vi "Control.vi"() -> ()   [LabVIEW 2024]
uses:
  <vilib>/Instr/_visa.llb/VISA Configure Serial Port (Instr).vi
panel:
  in  "OK Button":bool
  in  "Enter Speed":dbl(slide) scale=10.0..100.0
  in  "VISA resource name":refnum<visa-resource-name>
  in  "Stop Button":bool
  out "Boolean 4":bool
  out "Boolean 3":bool
  out "Boolean 2":bool
  out "Boolean":bool
  in  "Next Button":bool
  in  "Previous Button":bool
  in  "Down Button":bool
  in  "Up Button":bool
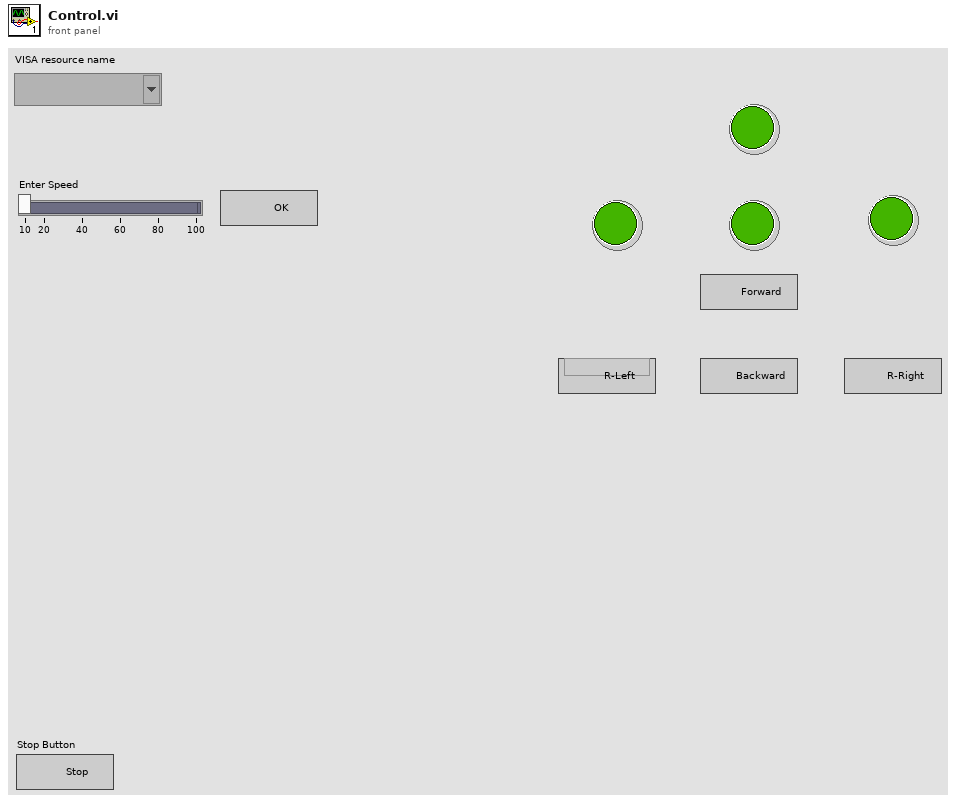
[diagram p1: front panel]
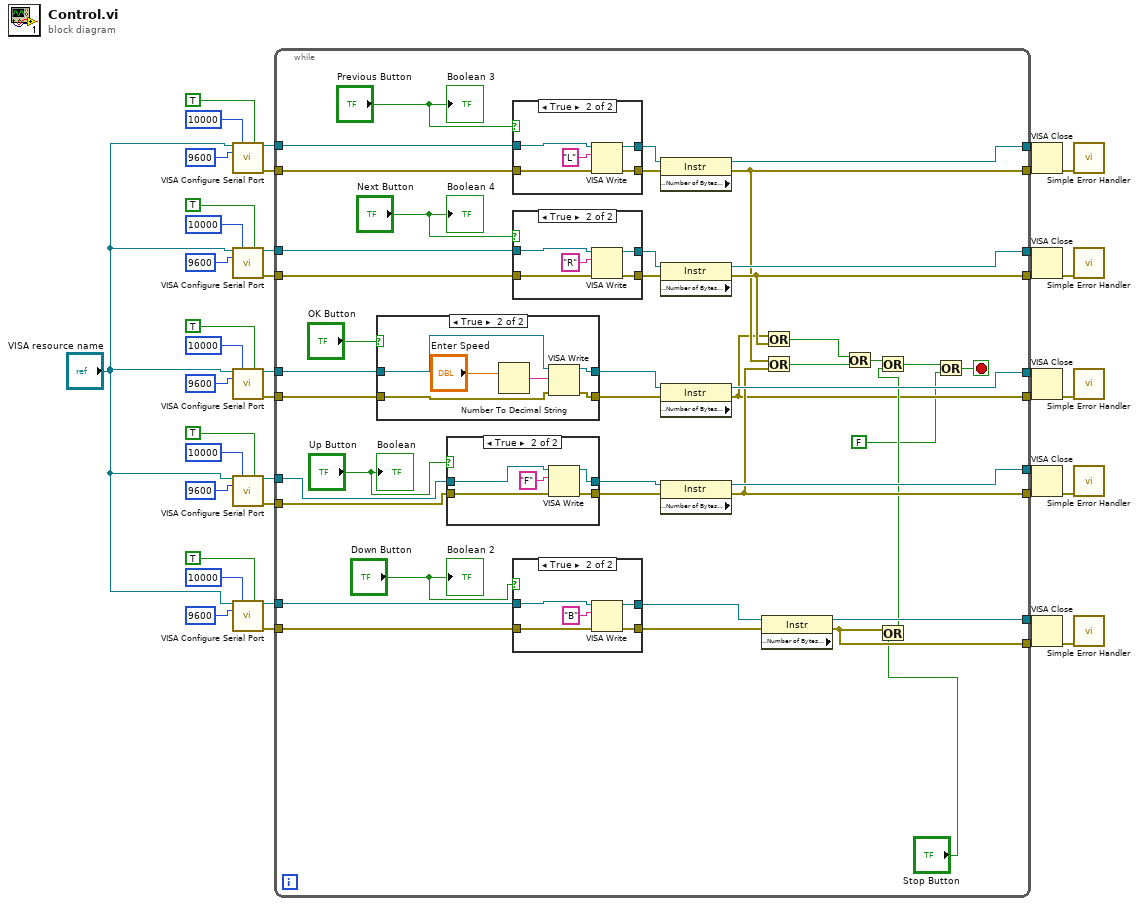
[diagram p0: block diagram]
diagram:
  n1 = call-poly "VISA Configure Serial Port"("VISA resource name"="VISA resource name", "timeout (10sec)"=10000, "Enable Termination\nChar (T)"=TRUE, "baud rate (9600)"=9600) -> ("VISA resource name out"=w22:refnum<visa-resource-name>, "error out"=w23:errorcluster)  [unwired: 10 in]
  n2 = call-poly "VISA Configure Serial Port"("VISA resource name"="VISA resource name", "timeout (10sec)"=10000, "Enable Termination\nChar (T)"=TRUE, "baud rate (9600)"=9600) -> ("VISA resource name out"=w26:refnum<visa-resource-name>, "error out"=w34:errorcluster)  [unwired: 10 in]
  n3 = call-poly "VISA Configure Serial Port"("VISA resource name"="VISA resource name", "timeout (10sec)"=10000, "Enable Termination\nChar (T)"=TRUE, "baud rate (9600)"=9600) -> ("VISA resource name out"=w41:refnum<visa-resource-name>, "error out"=w40:errorcluster)  [unwired: 10 in]
  n4 = call-poly "VISA Configure Serial Port"("VISA resource name"="VISA resource name", "timeout (10sec)"=10000, "Enable Termination\nChar (T)"=TRUE, "baud rate (9600)"=9600) -> ("VISA resource name out"=w14:refnum<visa-resource-name>, "error out"=w13:errorcluster)  [unwired: 10 in]
  n5 = call-poly "VISA Configure Serial Port"("VISA resource name"="VISA resource name", "timeout (10sec)"=10000, "Enable Termination\nChar (T)"=TRUE, "baud rate (9600)"=9600) -> ("VISA resource name out"=w3:refnum<visa-resource-name>, "error out"=w2:errorcluster)  [unwired: 10 in]
  n6 = while {
    tunnel: w41 -> [w84]
    tunnel: w40 -> [w83]
    tunnel: [w81] -> w39
    tunnel: [w44] -> w38
    tunnel: w34 -> [w75]
    tunnel: [w53] -> w33
    tunnel: [w74] -> w31
    tunnel: w26 -> [w73]
    tunnel: w23 -> [w69]
    tunnel: w22 -> [w68]
    tunnel: [w52] -> w19
    tunnel: [w66] -> w18
    tunnel: w14 -> [w63]
    tunnel: w13 -> [w62]
    tunnel: [w61] -> w11
    tunnel: [w51] -> w10
    tunnel: [w57] -> w5
    tunnel: [w50] -> w4
    tunnel: w3 -> [w56]
    tunnel: w2 -> [w55]
    stop <- w82 stop-if-true
    n7 = case shown="True" "OK Button" {
      tunnel: w84 -> [w113 w120]
      tunnel: w83 -> [w114 w119]
      tunnel: [w113 w118] -> w80
      tunnel: [w114 w117] -> w79
      frame False {
      }
      frame True {
        n8 = Number To Decimal String(number="Enter Speed") -> (decimal integer string=w115:string)  [unwired: 1 in]
        n9 = VISA Write(VISA resource name=w120, write buffer=w115, error in (no error)=w119) -> (VISA resource name out=w118:refnum<visa-resource-name>, error out=w117:errorcluster)  [unwired: 1 out]
      }
    }
    n10 = case shown="True" "Up Button" {
      tunnel: w63 -> [w92 w98]
      tunnel: w62 -> [w93 w97]
      tunnel: [w92 w96] -> w65
      tunnel: [w93 w95] -> w64
      frame False {
      }
      frame True {
        n11 = VISA Write(VISA resource name=w98, write buffer="F", error in (no error)=w97) -> (VISA resource name out=w96:refnum<visa-resource-name>, error out=w95:errorcluster)  [unwired: 1 out]
      }
    }
    n12 = case shown="True" "Previous Button" {
      tunnel: w68 -> [w99 w105]
      tunnel: w69 -> [w100 w104]
      tunnel: [w99 w103] -> w71
      tunnel: [w100 w102] -> w70
      frame False {
      }
      frame True {
        n13 = VISA Write(VISA resource name=w105, write buffer="L", error in (no error)=w104) -> (VISA resource name out=w103:refnum<visa-resource-name>, error out=w102:errorcluster)  [unwired: 1 out]
      }
    }
    n14 = case shown="True" "Next Button" {
      tunnel: w73 -> [w106 w112]
      tunnel: w75 -> [w107 w111]
      tunnel: [w106 w110] -> w77
      tunnel: [w107 w109] -> w76
      frame False {
      }
      frame True {
        n15 = VISA Write(VISA resource name=w112, write buffer="R", error in (no error)=w111) -> (VISA resource name out=w110:refnum<visa-resource-name>, error out=w109:errorcluster)  [unwired: 1 out]
      }
    }
    n16 = case shown="True" "Down Button" {
      tunnel: w56 -> [w85 w91]
      tunnel: w55 -> [w86 w90]
      tunnel: [w85 w89] -> w59
      tunnel: [w86 w88] -> w58
      frame False {
      }
      frame True {
        n17 = VISA Write(VISA resource name=w91, write buffer="B", error in (no error)=w90) -> (VISA resource name out=w89:refnum<visa-resource-name>, error out=w88:errorcluster)  [unwired: 1 out]
      }
    }
    n18 = property class="Instr" props=["Serial Settings:Number of Bytes at Serial Port"](reference=w71, error in=w70) -> (reference out=w66:refnum<visa-resource-name>, error out=w52:errorcluster)  [unwired: 1 out]
    n19 = property class="Instr" props=["Serial Settings:Number of Bytes at Serial Port"](reference=w77, error in=w76) -> (reference out=w74:refnum<visa-resource-name>, error out=w53:errorcluster)  [unwired: 1 out]
    n20 = property class="Instr" props=["Serial Settings:Number of Bytes at Serial Port"](reference=w80, error in=w79) -> (reference out=w81:refnum<visa-resource-name>, error out=w44:errorcluster)  [unwired: 1 out]
    n21 = property class="Instr" props=["Serial Settings:Number of Bytes at Serial Port"](reference=w65, error in=w64) -> (reference out=w61:refnum<visa-resource-name>, error out=w51:errorcluster)  [unwired: 1 out]
    n22 = property class="Instr" props=["Serial Settings:Number of Bytes at Serial Port"](reference=w59, error in=w58) -> (reference out=w57:refnum<visa-resource-name>, error out=w50:errorcluster)  [unwired: 1 out]
    n23 = Or(x=w44, y=w53) -> (x .or. y?=w49:bool)
    n24 = Or(x=w52, y=w51) -> (x .or. y?=w48:bool)
    n25 = Or(x=w49, y=w48) -> (x .or. y?=w47:bool)
    n26 = Or(x=w50, y="Stop Button") -> (x .or. y?=w46:bool)
    n27 = Or(x=w47, y=w46) -> (x .or. y?=w45:bool)
    n28 = Or(x=w45, y=FALSE) -> (x .or. y?=w82:bool)
    "Boolean 2" <- "Down Button"
    "Boolean" <- "Up Button"
    "Boolean 4" <- "Next Button"
    "Boolean 3" <- "Previous Button"
  }
  n29 = VISA Close(VISA resource name=w18, error in (no error)=w19) -> (error out=w20:errorcluster)
  n30 = VISA Close(VISA resource name=w31, error in (no error)=w33) -> (error out=w32:errorcluster)
  n31 = VISA Close(VISA resource name=w39, error in (no error)=w38) -> (error out=w37:errorcluster)
  n32 = VISA Close(VISA resource name=w11, error in (no error)=w10) -> (error out=w12:errorcluster)
  n33 = VISA Close(VISA resource name=w5, error in (no error)=w4) -> (error out=w6:errorcluster)
  n34 = call <vilib>:"Simple Error Handler.vi"("error in (no error)"=w20) -> ()  [unwired: 4 in, 5 out]
  n35 = call <vilib>:"Simple Error Handler.vi"("error in (no error)"=w32) -> ()  [unwired: 4 in, 5 out]
  n36 = call <vilib>:"Simple Error Handler.vi"("error in (no error)"=w37) -> ()  [unwired: 4 in, 5 out]
  n37 = call <vilib>:"Simple Error Handler.vi"("error in (no error)"=w12) -> ()  [unwired: 4 in, 5 out]
  n38 = call <vilib>:"Simple Error Handler.vi"("error in (no error)"=w6) -> ()  [unwired: 4 in, 5 out]
